vi "ErrorCheckHWI.vi"(8 "error in (no error)":errorcluster, 11 "DMD in":refnum<class "DMD.lvclass">) -> (0 "error out":errorcluster, 3 "DMD out":refnum<class "DMD.lvclass">)   [LabVIEW 2013, in "DMD.lvclass"]
uses:
  DMD.lvclass
  DMD.lvclass/DMD.ctl
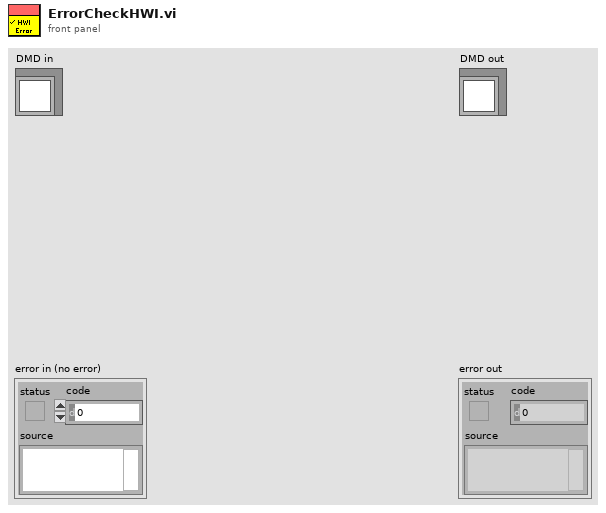
[diagram p1: front panel]
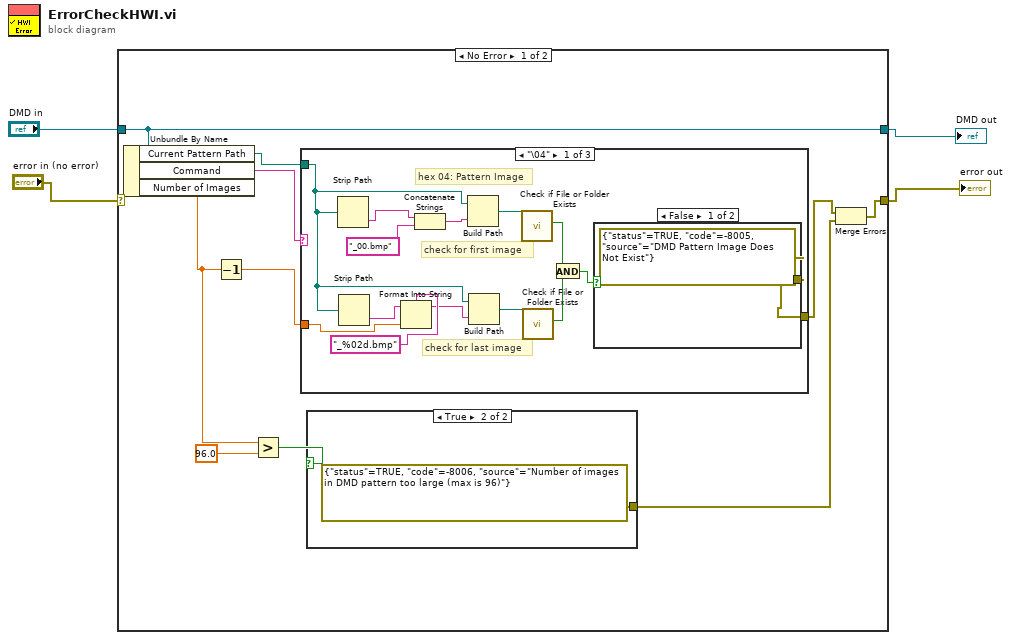
[diagram p0: block diagram]
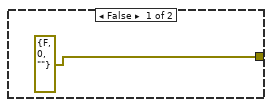
[diagram p2: hidden frame]
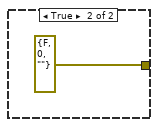
[diagram p3: hidden frame]
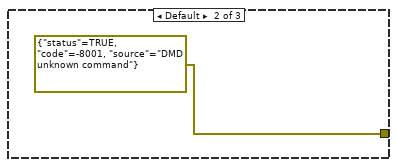
[diagram p4: hidden frame]
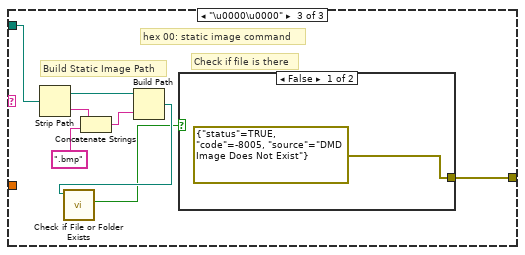
[diagram p5: hidden frame]
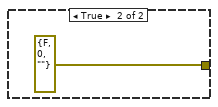
[diagram p6: hidden frame]
diagram:
  n1 = case shown="No Error" "error in (no error)" {
    selector: "error in (no error)" -> [_ w44]
    tunnel: "DMD in" -> [w14 w45]
    tunnel: [w14 w45] -> w2
    tunnel: [w5 w44] -> w1
    frame No Error {
      n2 = Unbundle By Name(w14) -> ("Current Pattern Path"=w12:path, "Command"=w13:string, "Number of Images"=w10:dbl)
      n3 = Decrement(x=w10) -> (x-1=w11:dbl)
      n4 = Greater?(x=w10, y=96.0) -> (0:w8:bool)
      n5 = case shown="\"\\04\"" w13 {
        tunnel: w12 -> [w25 _ w35]
        tunnel: [w18 errorcluster {"status"=TRUE, "code"=-8001, "source"="DMD unknown command"} ("error out") w34] -> w7
        tunnel: w11 -> [w22 _ _]
        frame "\u0004" {
          # "check for last image"
          # "check for first image"
          # "hex 04: Pattern Image"
          n6 = Strip Path(path=w25) -> (name=w30:string)  [unwired: 1 out]
          n7 = Strip Path(path=w25) -> (name=w24:string)  [unwired: 1 out]
          n8 = Format Into String(format string="_%02d.bmp" ("string"), initial string=w24, w22) -> (resulting string=w17:string)  [unwired: 1 in, 1 out]
          n9 = Concatenate Strings(w30, "_00.bmp" ("string")) -> (w28:string)
          n10 = Build Path(base path=w25, name or relative path=w28) -> (appended path=w27:path)
          n11 = Build Path(base path=w25, name or relative path=w17) -> (appended path=w26:path)
          n12 = call <vilib>:"Check if File or Folder Exists.vi"("path"=w27) -> ("file or folder exists?"=w20:bool)  [unwired: 8 in, 2 out]
          n13 = call <vilib>:"Check if File or Folder Exists.vi"("path"=w26) -> ("file or folder exists?"=w21:bool)  [unwired: 8 in, 2 out]
          n14 = And(x=w20, y=w21) -> (x .and. y?=w19:bool)
          n15 = case shown="False" w19 {
            tunnel: [errorcluster {"status"=TRUE, "code"=-8005, "source"="DMD Pattern Image Does Not Exist"} ("error out") errorcluster {"status"=FALSE, "code"=0, "source"=""} ("error out")] -> w18
            frame False {
            }
            frame True {
            }
          }
        }
        frame Default {
        }
        frame "\u0000\u0000" {
          # "Check if file is there"
          # "Build Static Image Path"
          # "hex 00: static image command"
          n16 = Strip Path(path=w35) -> (stripped path=w38:path, name=w41:string)
          n17 = Concatenate Strings(w41, ".bmp" ("string")) -> (w39:string)
          n18 = Build Path(base path=w38, name or relative path=w39) -> (appended path=w37:path)
          n19 = call <vilib>:"Check if File or Folder Exists.vi"("path"=w37) -> ("file or folder exists?"=w36:bool)  [unwired: 8 in, 2 out]
          n20 = case shown="False" w36 {
            tunnel: [errorcluster {"status"=TRUE, "code"=-8005, "source"="DMD Image Does Not Exist"} ("error out") errorcluster {"status"=FALSE, "code"=0, "source"=""} ("error out")] -> w34
            frame False {
            }
            frame True {
            }
          }
        }
      }
      n21 = case shown="True" w8 {
        tunnel: [errorcluster {"status"=FALSE, "code"=0, "source"=""} ("error out") errorcluster {"status"=TRUE, "code"=-8006, "source"="Number of images in DMD pattern too large (max is 96)"} ("error out")] -> w6
        frame False {
        }
        frame True {
        }
      }
      n22 = Merge Errors(w7, w6) -> (w5:errorcluster)
    }
    frame Error {
    }
  }
  "error out" <- w1
  "DMD out" <- w2
